vi "Overlay Pattern Matching Results (Single VI).vi"(6 "Color":u32(colorbox)=16711680, 7 "Group":string, 8 "error in":errorcluster, 10 "Matches":T2(array[cluster]), 11 "Image":T1) -> (0 "error out":errorcluster, 3 "Image Out":T1)   [LabVIEW 2014]
uses:
  <vilib>/vision/Image Controls.llb/IMAQ Image.ctl
panel:
  # "LICENSED MATERIALS – PROPERTY OF IBM\nCopyright IBM Corp. 2016,\nALL RIGHTS RESERVED"
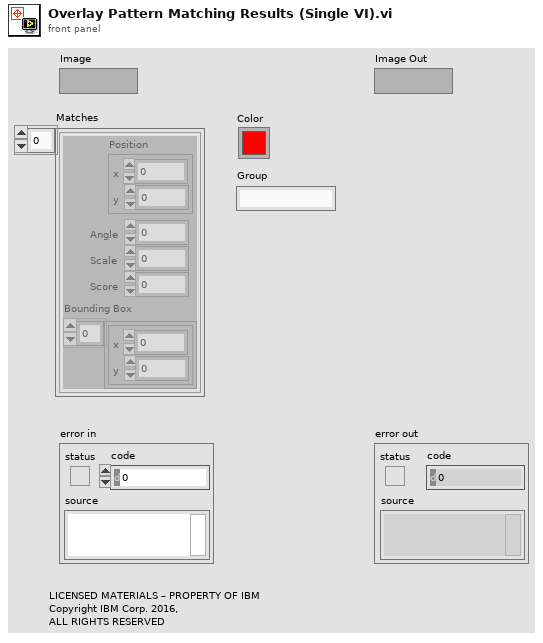
[diagram p1: front panel]
types:
  T1 = typedef "IMAQ Image.ctl" = refnum<image>
  T2 = cluster{"Position":cluster{"x":sgl, "y":sgl}, "Angle":sgl, "Scale":sgl, "Score":sgl, "Bounding Box":cluster{"x":sgl, "y":sgl}[]}[]
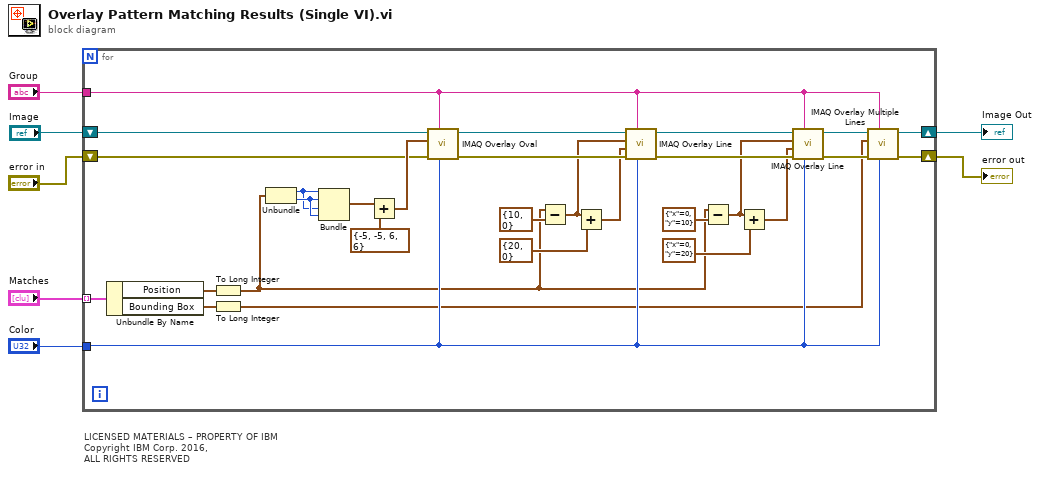
[diagram p0: block diagram]
diagram:
  # "LICENSED MATERIALS – PROPERTY OF IBM\nCopyright IBM Corp. 2016,\nALL RIGHTS RESERVED"
  n1 = for {
    shift-right: [w16] -> w6
    shift-left: "Image" -> [w21]
    tunnel: "Matches" -> [w37] mode=indexing
    tunnel: "Color" -> [w19]
    shift-right: [w15] -> w2
    shift-left: "error in" -> [w20]
    tunnel: "Group" -> [w22]
    n2 = Unbundle By Name(w37) -> ("Position"=w17:cluster{"x":sgl, "y":sgl}, "Bounding Box"=w18:cluster{"x":sgl, "y":sgl}[])
    n3 = To Long Integer(number=w17) -> (32bit integer=w12:cluster{"x":i32, "y":i32})
    n4 = To Long Integer(number=w18) -> (32bit integer=w14:cluster{"x":i32, "y":i32}[])
    n5 = Unbundle(w12) -> ("x"=w25:i32, "y"=w26:i32)
    n6 = Bundle("x"=w25, "y"=w26, "x"=w25, "y"=w26) -> (w13:cluster{"x":i32, "y":i32, "x":i32, "y":i32})  [unwired: 1 out]
    n7 = Add(x=w13, y=cluster{"y":i32, "x":i32, "y":i32, "x":i32} {"y"=-5, "x"=-5, "y"=6, "x"=6}) -> (x+y=w28:cluster{i32, i32, i32, i32})
    n8 = call "IMAQ Overlay Oval"("Color"=w19, "Group"=w22, "error in (no error)"=w20, "Bounding Rectangle"=w28, "Image"=w21) -> ("error out"=w34:errorcluster, "Image Out"=w23:T1)  [unwired: 1 in, 4 out]
    n9 = Subtract(x=w12, y=cluster{"x":i32, "y":i32} {"x"=10, "y"=0}) -> (x-y=w11:cluster{"x":i32, "y":i32})
    n10 = Add(x=w11, y=cluster{"x":i32, "y":i32} {"x"=20, "y"=0}) -> (x+y=w8:cluster{"x":i32, "y":i32})
    n11 = call "IMAQ Overlay Line"("Color"=w19, "Group"=w22, "error in (no error)"=w34, "End Point"=w8, "Start Point"=w11, "Image"=w23) -> ("error out"=w35:errorcluster, "Image Out"=w33:T1)  [unwired: 4 out]
    n12 = Subtract(x=w12, y=cluster{"x":i32, "y":i32} {"x"=0, "y"=10}) -> (x-y=w10:cluster{"x":i32, "y":i32})
    n13 = Add(x=w10, y=cluster{"x":i32, "y":i32} {"x"=0, "y"=20}) -> (x+y=w9:cluster{"x":i32, "y":i32})
    n14 = call "IMAQ Overlay Line"("Color"=w19, "Group"=w22, "error in (no error)"=w35, "End Point"=w9, "Start Point"=w10, "Image"=w33) -> ("error out"=w36:errorcluster, "Image Out"=w24:T1)  [unwired: 4 out]
    n15 = call "IMAQ Overlay Multiple Lines"("Color"=w19, "Group"=w22, "error in (no error)"=w36, "Line End Points"=w14, "Image"=w24) -> ("error out"=w15:errorcluster, "Image Out"=w16:T1)  [unwired: 1 in, 4 out]
  }
  "Image Out" <- w6
  "error out" <- w2
